vi "Build Last Error Info.vi"(8 "error in (no error)":errorcluster, 10 "error code in":i32, 11 "handle in":u64) -> (0 "error out":errorcluster, 1 "error info":T1 items=["ERRINFO_ERROR", "ERRINFO_WARNING", "ERRINFO_INFO"], 2 "error code out":i32, 3 "handle out":u64, 5 "error string out":string)   [LabVIEW 2020, in "Ballard ARINC 429 Hardware API.lvlib"]
doc: "Builds an error string based on the last error encountered by the device associated with <B>handle in </B>. If no handle is provided, this VI will produce the error string associated with <B>error code in </B> and translate to the LabVIEW error code contained in <B>error code out</B>."
uses:
  <instrlib>/BTICardLib/Public/Controls/Error Info.ctl
  Ballard ARINC 429 Hardware API.lvlib
  BTICardLV.dll
  <instrlib>/BTICardLib/BTICardLV.lvlib
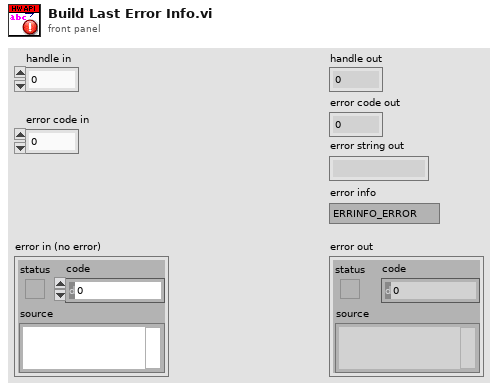
[diagram p1: front panel]
types:
  T1 = typedef "BTICardLV.lvlib/Error Info.ctl" = u32
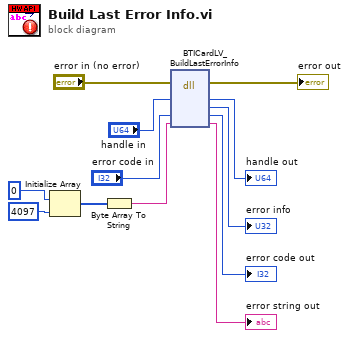
[diagram p0: block diagram]
diagram:
  n1 = Initialize Array(u8 0 ("element"), 4097 ("dimension size")) -> (w7:u8[])
  n2 = Byte Array To String(unsigned byte array=w7) -> (string=w6:string)
  n3 = dll-call lib="BTICardLV.*" fn="BTICardLV_BuildLastErrorInfo"(error in="error in (no error)", "handle"="handle in", "errorinout"="error code in", "errorstringout"=w6) -> (error out=→"error out":errorcluster, "handle"=→"handle out":u64, "outinfo"=→"error info":u32, "errorinout"=→"error code out":i32, "errorstringout"=→"error string out":string)  [unwired: 4 in, 1 out]
